vi "Handle Remote Command.vi"(8 "error in (no error)":errorcluster, 9 "Data":string, 10 "Command":string, 11 "Example Instrument in":refnum<class "Example Instrument.lvclass">) -> (0 "error out":errorcluster, 2 "Variant":variant, 3 "Example Instrument out":refnum<class "Example Instrument.lvclass">)   [LabVIEW 2016, in "Example Instrument.lvclass"]
uses:
  Example Instrument.lvclass
  Instrument.lvclass
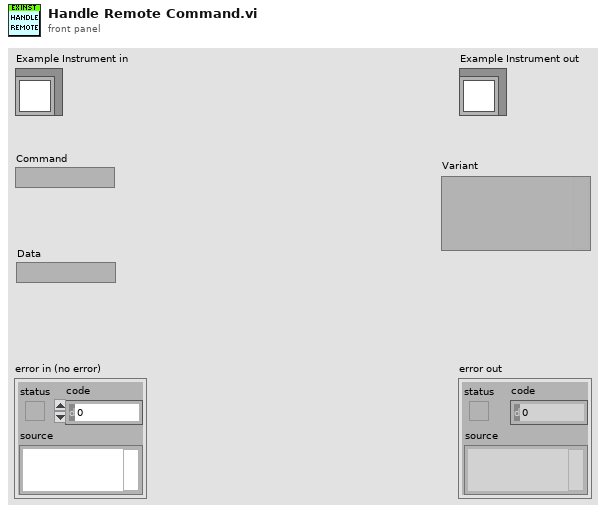
[diagram p1: front panel]
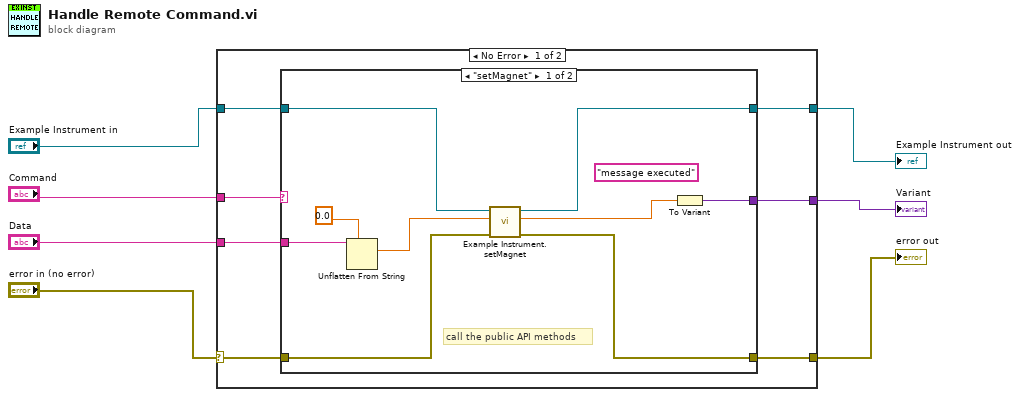
[diagram p0: block diagram]
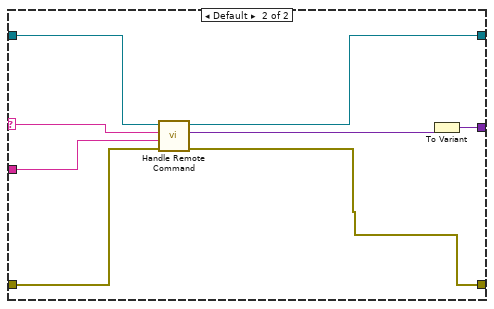
[diagram p2: hidden frame]
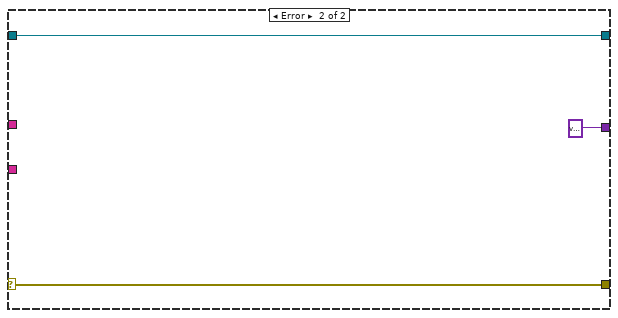
[diagram p3: hidden frame]
diagram:
  n1 = case shown="No Error" "error in (no error)" {
    selector: "error in (no error)" -> [w10 w34]
    tunnel: [w9 w34] -> w4
    tunnel: [w12 w33] -> w2
    tunnel: "Example Instrument in" -> [w13 w33]
    tunnel: "Command" -> [w14 _]
    tunnel: [w11 variant ("Variant")] -> w3
    tunnel: "Data" -> [w8 _]
    frame No Error {
      n2 = case shown="\"setMagnet\"" w14 {
        selector: w14 -> [_ w29]
        tunnel: w13 -> [w22 w25]
        tunnel: [w21 w24] -> w12
        tunnel: [w23 w31] -> w11
        tunnel: w10 -> [w20 w27]
        tunnel: [w19 w26] -> w9
        tunnel: w8 -> [w18 w28]
        frame "setMagnet" {
          (unwired) "message executed"
          # "call the public API methods"
          n3 = Unflatten From String(type=0.0, binary string=w18) -> (value=w16:dbl)  [unwired: 3 in, 2 out]
          n4 = call "Example Instrument.setMagnet.vi"("error in (no error)"=w20, "setMagnet"=w16, "Example Instrument"=w22) -> ("error out"=w19:errorcluster, "notification"=w15:dbl, "Example Instrument out"=w21:refnum<class "Example Instrument.lvclass">)  [unwired: 5 in, 1 out]
          n5 = To Variant(anything=w15) -> (Variant=w23:variant)
        }
        frame Default {
          n6 = call-parent "Handle Remote Command.vi"("error in (no error)"=w27, "Data"=w28, "Command"=w29, "Instrument in"=w25) -> ("error out"=w26:errorcluster, "Variant"=w30:variant, "Instrument out"=w24:refnum<class "Example Instrument.lvclass">)  [unwired: 5 in]
          n7 = To Variant(anything=w30) -> (Variant=w31:variant)
        }
      }
    }
    frame Error {
    }
  }
  "error out" <- w4
  "Example Instrument out" <- w2
  "Variant" <- w3
